vi "Peak Detection in a Signal with Baseline Wandering.vi"() -> ()   [LabVIEW 2023]
doc: "This example demonstrates how to use the WA Multiscale Peak Detection VI to detect peaks in ECG signals. Typically, ECG signals contain baseline wandering. Therefore, the heartbeats (peaks) in ECG signals can be difficult to detect by using a fixed threshold. The WA Multiscale Peak Detection VI enables you to specify <b>Threshold</b>, <b>Width</b>, and <b>Detrend Settings</b> to detect the heartbeats in ECG signals.\n\n<b>Instructions:</b>\n1. Run this VI.\n2. Change <b>Threshold</b>, <b>Width</b>, and <b>Detrend Settings</b>.\n3. Observe the different results."
uses:
  <vilib>/addons/Wavelet Analysis/application.llb/WA Multiscale Peak Detection (Waveform).vi
  <vilib>/addons/_Advanced Signal Processing/NI_AdvSigProcWA.lvlib
panel:
  out "Peak Plot":cluster{"Ramp Pattern":dbl[], "X":dbl[]}[](graph)
  in  "Detrend settings":cluster{"Detrend?":bool, "Trend frequency":dbl}={"Detrend?"=TRUE, "Trend frequency"=0.5} {"Trend frequency" step=0.1}
  in  "Width":i32=8
  in  "Threshold":dbl=0.4 min=-1.0 max=1.0
  in  "Stop":bool
  # "Overview: Demonstrates how to use the WA Multiscale Peak Detection VI to detect peaks in ECG signals. \nRequirements: LabVIEW Full Development System, Advanced Signal Processing Toolkit\nInstructions: \n1. Run this VI.\n2. Change Threshold, Width, and Detrend Settings.\n3. Observe the different results.\n4. Click Stop to stop the VI."
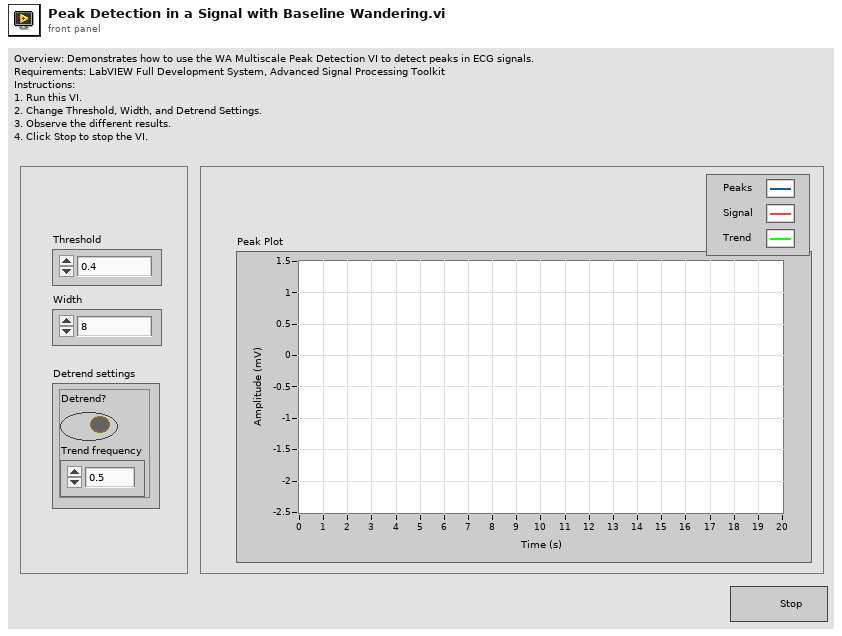
[diagram p1: front panel]
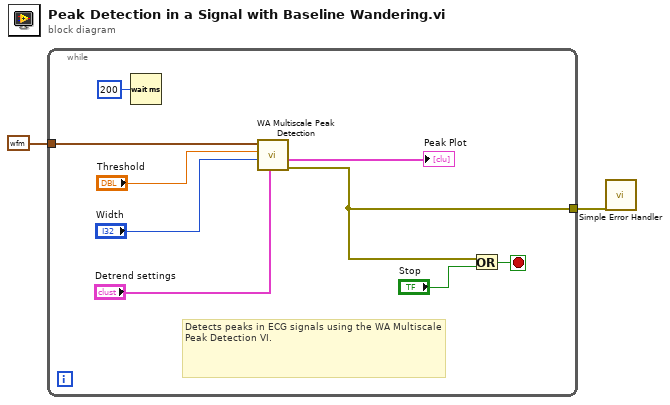
[diagram p0: block diagram]
diagram:
  n1 = while {
    tunnel: waveform(dbl) {"t0"=timestamp(-126126000 s since 1904-01-01), "dt"=0.004, "Y"=array[5000 elements]} ("Waveform Graph") -> [w10]
    tunnel: [w5] -> w1
    stop <- w3 stop-if-true
    # "Detects peaks in ECG signals using the WA Multiscale Peak Detection VI."
    n2 = Wait (ms)(milliseconds to wait=u32 200 ("millisecond multiple")) -> ()  [unwired: 1 out]
    n3 = call-poly <vilib>:"WA Multiscale Peak Detection.vi"("detrend settings"="Detrend settings", "width"="Width", "threshold"="Threshold", "signal"=w10) -> ("error out"=w5:errorcluster, "peak plot"=→"Peak Plot":cluster{"Ramp Pattern":dbl[], "X":dbl[]}[])  [unwired: 3 in, 3 out]
    n4 = Or(x=w5, y="Stop") -> (x .or. y?=w3:bool)
  }
  n5 = call <vilib>:"Simple Error Handler.vi"("error in (no error)"=w1) -> ()  [unwired: 4 in, 5 out]
